vi "Do.vi"(8 "error in (no error)":errorcluster, 10 "Actor in":refnum<class "Actor.lvclass">, 11 "Set Mixer Msg in":refnum<class "Set Mixer Msg.lvclass">) -> (0 "error out":errorcluster, 2 "Actor out":refnum<class "Actor.lvclass">)   [LabVIEW 2018, in "Feeder Actor.lvlib" / "Set Mixer Msg.lvclass"]
doc: "(<B>Filename</B>: Actor Framework.lvlib:Message.lvclass:Do.vi)\n\nDefines what a message does when it is received by an actor. Generally, a message instructs an actor to invoke one of its methods. By default, this method does nothing. A child class must override it to define behavior. Create a child class by using the Actor Framework Message Maker dialog box."
uses:
  Set Mixer Msg.lvclass
  <vilib>/ActorFramework/Actor/Actor.lvclass
  Mixer/Mixer.lvclass
  C:/Program Files/National Instruments/LabVIEW 2018/vi.lib/ActorFramework/Actor/Actor.lvclass
  Set Mixer Msg.lvclass/Set Mixer Msg.ctl
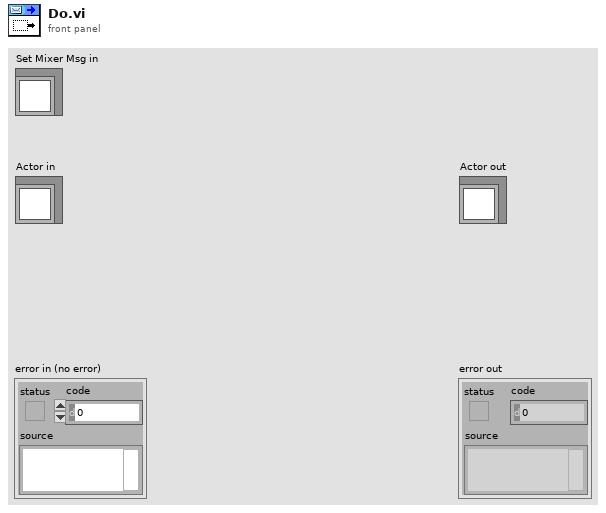
[diagram p1: front panel]
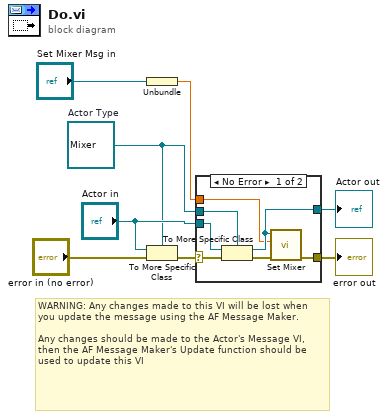
[diagram p0: block diagram]
diagram:
  w3 = refnum<class "Mixer.lvclass"> refnum  # Actor Type
  # "WARNING: Any changes made to this VI will be lost when you update the message using the AF Message Maker.\n\nAny changes should be made to the Actor's Message VI, then the AF Message Maker's Update function should be used to update this VI"
  n1 = Unbundle("Set Mixer Msg in") -> (w2:dbl)
  n2 = To More Specific Class(target class=w3, reference="Actor in", error in="error in (no error)") -> (error out=w7:errorcluster)  [unwired: 1 out]
  n3 = case shown="No Error" w7 {
    selector: w7 -> [w15 w17]
    tunnel: [w10 w17] -> w6
    tunnel: [w12 w16] -> w5
    tunnel: "Actor in" -> [w14 w16]
    tunnel: w3 -> [w13 _]
    tunnel: w2 -> [w9 _]
    frame No Error {
      n4 = To More Specific Class ("Actor Cast")(target class=w13, reference=w14, error in=w15) -> (specific class reference=w12:refnum<class "Mixer.lvclass">, error out=w11:errorcluster)
      n5 = call "Set Mixer.vi"("error in (no error)"=w11, "Mixer"=w9, "Feeder Actor.lvlib:Mixer.lvclass"=w12) -> ("error out"=w10:errorcluster)  [unwired: 7 in, 1 out]
    }
    frame Error {
    }
  }
  "error out" <- w6
  "Actor out" <- w5
